vi "CRYALL Resample.vi"(8 "error in (no error)":errorcluster, 9 "config":T1={"new sample period"=0.0, "Timing Jitter"=enum."Interpolation", "first point location"=0.0, "prototype filter"={"h"=[], "Max Decimation"=1000}} {"prototype filter"."h" format="%.2f"; "first point location" format="%.2f"; "new sample period" format="%.2f"}, 10 "anti-aliasing?":bool=TRUE, 11 "length of X":i32) -> (0 "error out":errorcluster, 1 "length of Y (after padding zeroes)":i32, 2 "length of Y":i32, 3 "length of padding zeroes":i32)   [LabVIEW 2013]
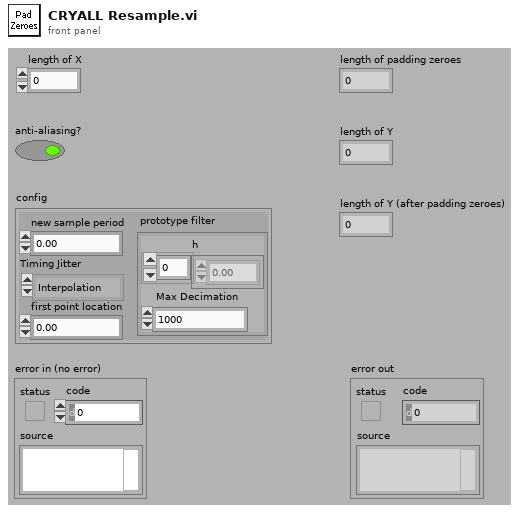
[diagram p1: front panel]
types:
  T1 = cluster{"new sample period":dbl, "Timing Jitter":enum32{"Interpolation", "Rounding"}, "first point location":dbl, "prototype filter":cluster{"h":dbl[], "Max Decimation":i32}}
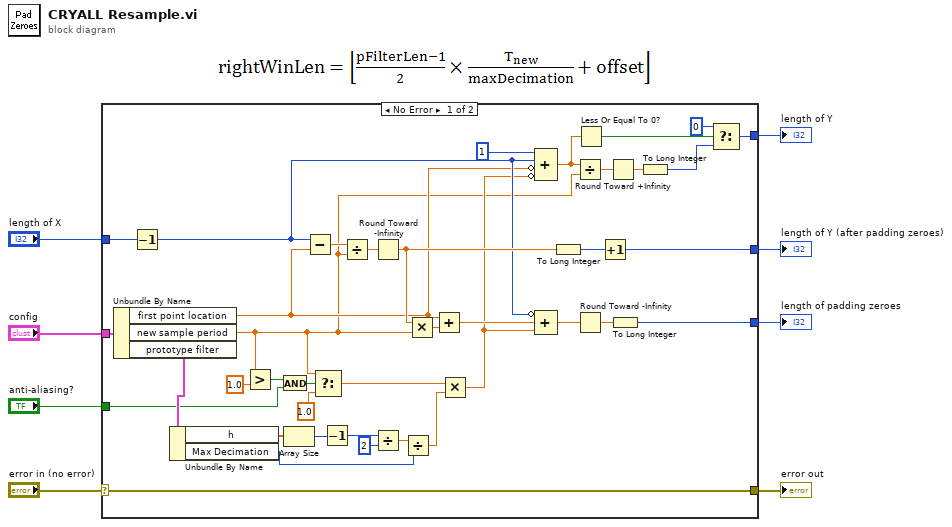
[diagram p0: block diagram]
diagram:
  n1 = case shown="No Error" "error in (no error)" {
    selector: "error in (no error)" -> [w25 w48]
    tunnel: "config" -> [w47 _]
    tunnel: [w33 _] -> w7
    tunnel: "length of X" -> [w28 _]
    tunnel: "anti-aliasing?" -> [w27 _]
    tunnel: [w25 w48] -> w3
    tunnel: [w22 _] -> w2
    tunnel: [w14 _] -> w1
    frame No Error {
      n2 = Unbundle By Name(w47) -> ("first point location"=w19:dbl, "new sample period"=w17:dbl, "prototype filter"=w43:cluster{"h":dbl[], "Max Decimation":i32})
      n3 = Decrement(x=w28) -> (x-1=w20:i32)
      n4 = Unbundle By Name(w43) -> ("h"=w42:dbl[], "Max Decimation"=w37:i32)
      n5 = Greater?(x=w17, y=1.0) -> (0:w26:bool)
      n6 = And(x=w26, y=w27) -> (x .and. y?=w31:bool)
      n7 = Array Size(array=w42) -> (size(s)=w41:i32)
      n8 = Subtract(x=w20, y=w19) -> (x-y=w46:dbl)
      n9 = Select(t=w17, s=w31, f=1.0) -> (s? t:f=w29:dbl)
      n10 = Decrement(x=w41) -> (x-1=w40:i32)
      n11 = Divide(x=w46, y=w17) -> (x/y=w45:dbl)
      n12 = Round Toward -Infinity(1:w45) -> (0:w21:dbl)
      n13 = Divide(x=w40, y=2) -> (x/y=w38:dbl)
      n14 = Divide(x=w38, y=w37) -> (x/y=w36:dbl)
      n15 = Multiply(x=w21, y=w17) -> (x*y=w44:dbl)
      n16 = Add(x=w19, y=w44) -> (x+y=w24:dbl)
      n17 = Multiply(x=w29, y=w36) -> (x*y=w18:dbl)
      n18 = Compound Arithmetic op=ADD(1 ("value"), w20, invert w19, invert w18) -> (w13:dbl)
      n19 = Compound Arithmetic op=ADD(invert w20, w24, w18) -> (w35:dbl)
      n20 = To Long Integer(number=w21) -> (32bit integer=w23:i32)
      n21 = Divide(x=w13, y=w17) -> (x/y=w11:dbl)
      n22 = Round Toward -Infinity(1:w35) -> (0:w34:dbl)
      n23 = Less Or Equal To 0?(x=w13) -> (x <= 0?=w16:bool)
      n24 = Increment(x=w23) -> (x+1=w22:i32)
      n25 = Round Toward +Infinity(x=w11) -> (ceil(x): smallest int >= x=w12:dbl)
      n26 = To Long Integer(number=w34) -> (32bit integer=w33:i32)
      n27 = To Long Integer(number=w12) -> (32bit integer=w10:i32)
      n28 = Select(t=0, s=w16, f=w10) -> (s? t:f=w14:i32)
    }
    frame Error {
    }
  }
  "error out" <- w3
  "length of padding zeroes" <- w7
  "length of Y (after padding zeroes)" <- w2
  "length of Y" <- w1
